vi "SweepDataPointsCheck_ver1.0.vi"(2 "Input # of sweep steps:":u32=100 step=1, 3 "Input # of total points:":u32=100 step=1) -> (0 "Output # of sweep steps:":u32=100 step=1, 1 "Output # of total points:":u32=100 step=1)   [LabVIEW 2012]
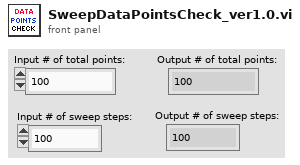
[diagram p1: front panel]
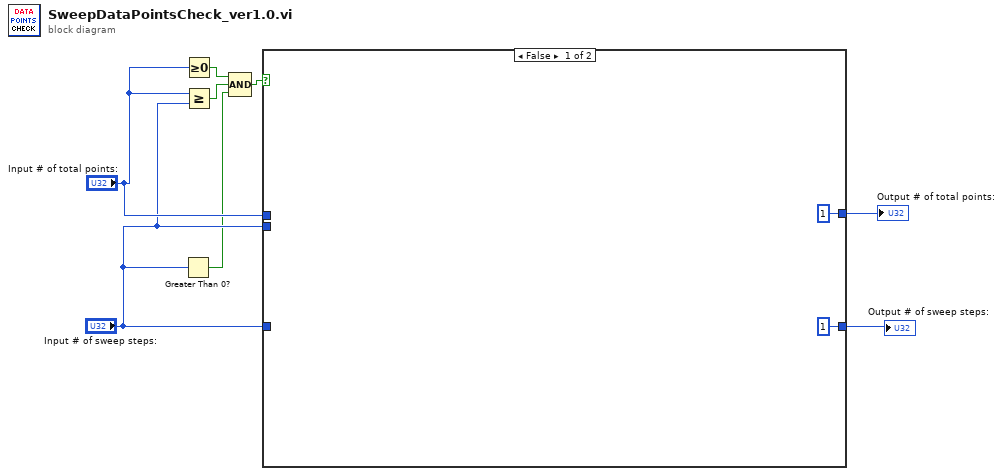
[diagram p0: block diagram]
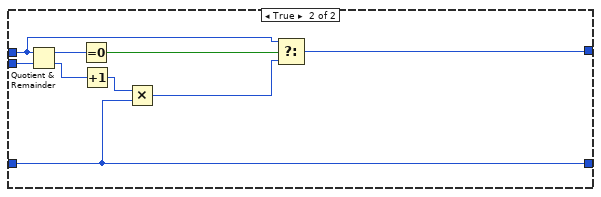
[diagram p2: hidden frame]
diagram:
  n1 = Greater Than 0?(x="Input # of sweep steps:") -> (x > 0?=w1:bool)
  n2 = Greater Or Equal To 0?(x="Input # of total points:") -> (x >= 0?=w6:bool)
  n3 = Greater Or Equal?(x="Input # of total points:", y="Input # of sweep steps:") -> (x >= y?=w5:bool)
  n4 = Compound Arithmetic op=AND(w6, w5, w1) -> (w7:bool)
  n5 = case shown="False" w7 {
    tunnel: "Input # of total points:" -> [_ w11]
    tunnel: "Input # of sweep steps:" -> [_ w17]
    tunnel: [u32 1 w16] -> w4
    tunnel: "Input # of sweep steps:" -> [_ w13]
    tunnel: [u32 1 ("Input # of sweep steps:") w13] -> w3
    frame False {
    }
    frame True {
      n6 = Quotient & Remainder(x=w11, y=w17) -> (x-y*floor(x/y)=w18:u32, floor(x/y)=w15:u32)
      n7 = Equal To 0?(x=w18) -> (x = 0?=w19:bool)
      n8 = Increment(x=w15) -> (x+1=w14:u32)
      n9 = Multiply(x=w14, y=w13) -> (x*y=w12:u32)
      n10 = Select(t=w11, s=w19, f=w12) -> (s? t:f=w16:u32)
    }
  }
  "Output # of sweep steps:" <- w3
  "Output # of total points:" <- w4
